vi "Configure Spurious Emission (Segment Level Setup).vi"(0 "VISA resource name":refnum<visa-resource-name>, 1 "Enable Preamp State (F:Disable)":bool, 5 "Spurious Reference Level":dbl[](array[numeric]) min=-120.0 max=50.0 format="%.2f", 7 "Spurious Attenuator":i32[](array[ring]) items=["Auto", "0 dB", "2 dB", "4 dB", "6 dB", "8 dB", "10 dB", "12 dB", "14 dB", "16 dB", "18 dB", "20 dB", "22 dB", "24 dB", "26 dB", "28 dB", "30 dB", "32 dB", "34 dB", "36 dB", "38 dB", "40 dB", "42 dB", "44 dB", "46 dB", "48 dB", "50 dB", "52 dB", "54 dB", "56 dB", "58 dB", "60 dB"], 9 "Spurious Preamp":i32[](array[ring]) items=["Off", "On"], 11 "error in (no error)":errorcluster) -> (4 "VISA resource name out":refnum<visa-resource-name>, 15 "error out":errorcluster)   [LabVIEW 2020, in "Anritsu Signal Analyzer Series.lvlib"]
doc: "Configures the level for segment parameter of Spurious Emission measurement."
uses:
  Anritsu Signal Analyzer Series.lvlib
panel:
  # "dBm"
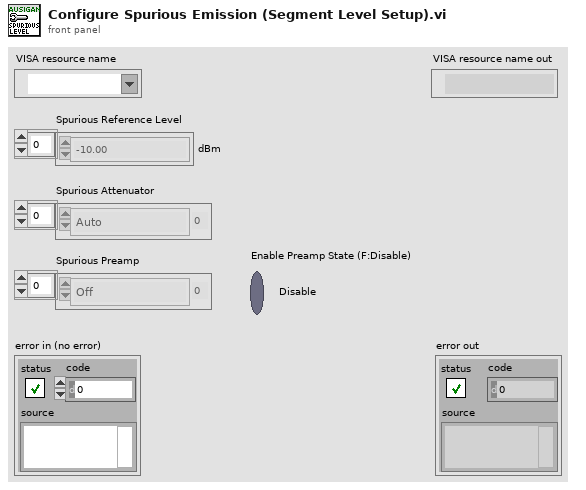
[diagram p1: front panel]
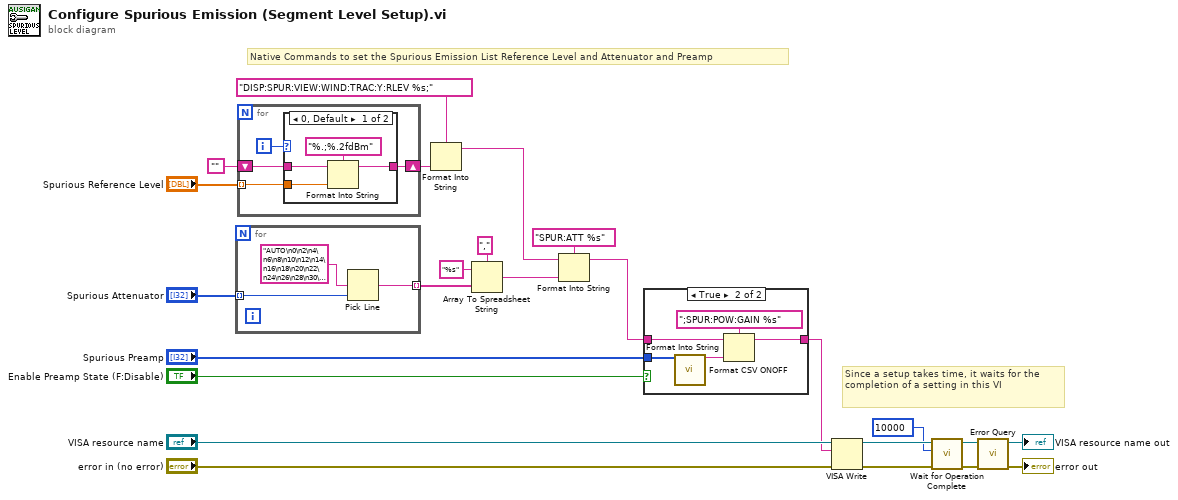
[diagram p0: block diagram]
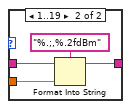
[diagram p2: hidden frame]
diagram:
  # "Since a setup takes time, it waits for the completion of a setting in this VI"
  # "Native Commands to set the Spurious Emission List Reference Level and Attenuator and Preamp"
  n1 = for {
    tunnel: "Spurious Attenuator" -> [w25] mode=indexing
    tunnel: [w26] -> w13 mode=indexing
    n2 = Pick Line(multi-line string="AUTO\n0\n2\n4\n6\n8\n10\n12\n14\n16\n18\n20\n22\n24\n26\n28\n30\n32\n34\n36\n38\n40\n42\n44\n46\n48\n50\n52\n54\n56\n58\n60" ("文字列"), line index=w25) -> (output string=w26:string)  [unwired: 1 in]
  }
  n3 = for {
    shift-right: [w28] -> w6
    shift-left: "" -> [w30]
    tunnel: "Spurious Reference Level" -> [w29] mode=indexing
    i -> [w31]
    n4 = case shown="0, Default" w31 {
      tunnel: w30 -> [w34 w37]
      tunnel: [w32 w36] -> w28
      tunnel: w29 -> [w33 w38]
      frame 0, Default {
        n5 = Format Into String(format string="%.;%.2fdBm" ("string"), initial string=w34, w33) -> (resulting string=w32:string)  [unwired: 1 in, 1 out]
      }
      frame 1..19 {
        n6 = Format Into String(format string="%.;,%.2fdBm" ("string"), initial string=w37, w38) -> (resulting string=w36:string)  [unwired: 1 in, 1 out]
      }
    }
  }
  n7 = Format Into String(format string="DISP:SPUR:VIEW:WIND:TRAC:Y:RLEV %s;" ("_CommandSet"), w6) -> (resulting string=w11:string)  [unwired: 2 in, 1 out]
  n8 = Array To Spreadsheet String(delimiter (Tab)=",", array=w13, 3:"%s" ("format string")) -> (spreadsheet string=w12:string)
  n9 = Format Into String(format string="SPUR:ATT %s" ("_CommandSet"), initial string=w11, w12) -> (resulting string=w9:string)  [unwired: 1 in, 1 out]
  n10 = case shown="True" "Enable Preamp State (F:Disable)" {
    tunnel: w9 -> [w40 w44]
    tunnel: [w40 w43] -> w8
    tunnel: "Spurious Preamp" -> [_ w42]
    frame False {
    }
    frame True {
      n11 = call "Format CSV ONOFF.vi"("Data_In"=w42) -> ("Data_out"=w41:string)  [unwired: 14 in]
      n12 = Format Into String(format string=";SPUR:POW:GAIN %s" ("_CommandSet"), initial string=w44, w41) -> (resulting string=w43:string)  [unwired: 1 in, 1 out]
    }
  }
  n13 = VISA Write(VISA resource name="VISA resource name", write buffer=w8, error in (no error)="error in (no error)") -> (VISA resource name out=w3:refnum<visa-resource-name>, error out=w2:errorcluster)  [unwired: 1 out]
  n14 = call "Wait for Operation Complete.vi"("error in (no error)"=w2, "Maximum Time (10000mSec)"=10000, "VISA resource name"=w3) -> ("error out"=w4:errorcluster, "VISA resource name out"=w5:refnum<visa-resource-name>)  [unwired: 7 in]
  n15 = call "Error Query.vi"("error in (no error)"=w4, "VISA resource name"=w5) -> ("error out"=→"error out":errorcluster, "VISA resource name out"=→"VISA resource name out":refnum<visa-resource-name>)  [unwired: 6 in, 2 out]
